vi "Test SFOAE Concurrent Stimuli.vi"() -> ()   [LabVIEW 2015]
uses:
  Typedefs/SFOAE-Stimulus Parameters.ctl
  Typedefs/SFOAE-Sweep Params.ctl
  <vilib>/Analysis/4window.llb/windowTd.ctl
  Utility VIs/Math VIs/FFT x(t) to dB,Degrees (1D).vi
  <vilib>/Analysis/NI_AALPro.lvlib
panel:
  out "Phase":cluster{"Array":dbl[], "Array":dbl[]}[](graph)
  out "Magnitude spectrum":cluster{"Array":dbl[], "Array":dbl[]}[](graph)
  in  "Cal File":path=path "C:/Experiment VIs/Cochlear Function Test Suite/LV Source/SFOAE VIs/Test VIs/dummy.calib"
  out "Waveform Graph":dbl[][](graph)
  in  "Fs (Hz)":dbl=100000.0
  in  "SFOAE Stim":T1={"Ear"=enum."Right", "Sweep"={"Type"=enum."Linear", "Fmin (kHz)"=4.0, "Fmax (kHz)"=14.25, "Rate"=5.0, "Ramp (ms)"=5.0, "Drain (ms)"=20.0}, "Suppressor"={"Delta"=50.0, "Ratio"=0.0, "Use ratio"=FALSE}, "Concurrent"={"Nsweeps"=1, "Overlap"=0.0}, "Ls (dB SPL)"=-23.0, "Lp (dB SPL)"={"Min"=-20.0, "Max"=-20.0, "Step"=5.0}}
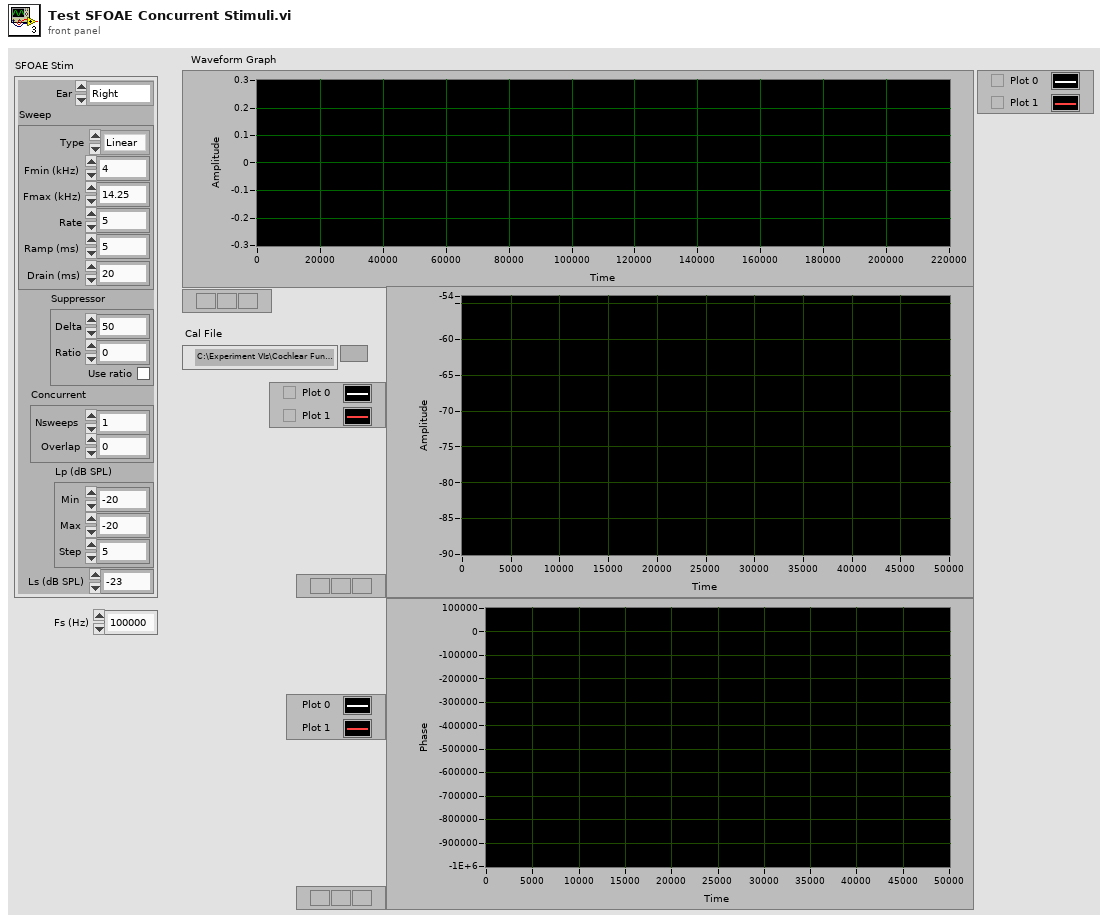
[diagram p1: front panel]
types:
  T1 = typedef "SFOAE-Stimulus Parameters.ctl" = cluster{"Ear":enum16{"Right", "Left"}, "Sweep":T2, "Suppressor":cluster{"Delta":dbl, "Ratio":dbl, "Use ratio":bool}, "Concurrent":cluster{"Nsweeps":i32, "Overlap":dbl}, "Ls (dB SPL)":dbl, "Lp (dB SPL)":cluster{"Min":dbl, "Max":dbl, "Step":dbl}}
  T2 = typedef "SFOAE-Sweep Params.ctl" = cluster{"Type":enum16{"Linear", "Log"}, "Fmin (kHz)":dbl, "Fmax (kHz)":dbl, "Rate":dbl, "Ramp (ms)":dbl, "Drain (ms)":dbl}
  T3 = typedef "NI_AALPro.lvlib/windowTd.ctl" = u32
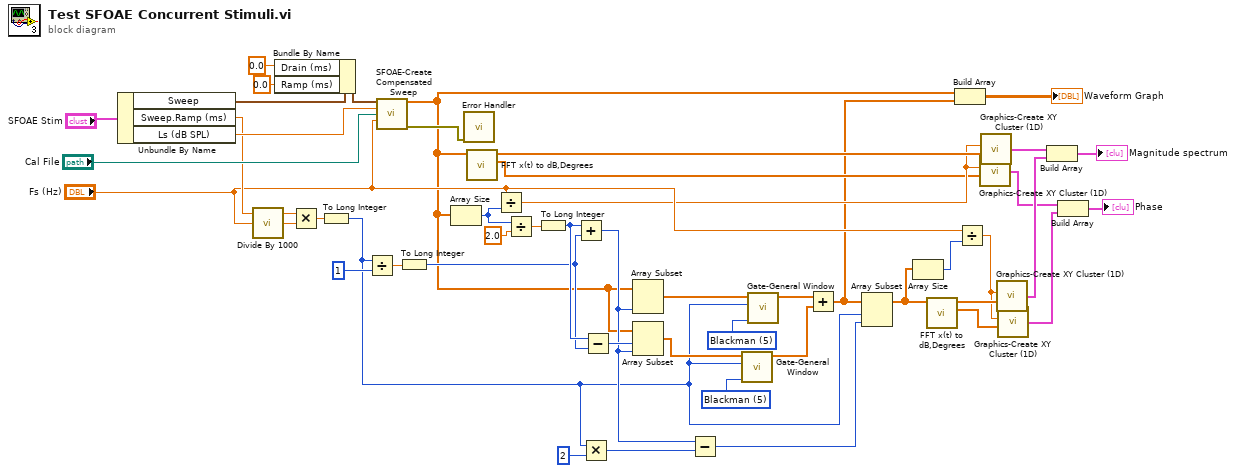
[diagram p0: block diagram]
diagram:
  w27 = T3 5 items=["Rectangle"=0, "Hanning"=1, "Hamming"=2, "Blackman-Harris"=3, "Exact Blackman"=4, "Blackman"=5, "Flat Top"=6, "4 Term B-Harris "=7, "7 Term B-Harris"=8, "Low Sidelobe"=9, "Blackman Nuttall"=11, "Triangle"=30, "Bartlett-Hanning"=31, "Bohman"=32, "Parzen"=33, "Welch"=34, "Kaiser"=60, "Dolph-Chebyshev"=61, "Gaussian"=62] ("window")
  w38 = T3 5 items=["Rectangle"=0, "Hanning"=1, "Hamming"=2, "Blackman-Harris"=3, "Exact Blackman"=4, "Blackman"=5, "Flat Top"=6, "4 Term B-Harris "=7, "7 Term B-Harris"=8, "Low Sidelobe"=9, "Blackman Nuttall"=11, "Triangle"=30, "Bartlett-Hanning"=31, "Bohman"=32, "Parzen"=33, "Welch"=34, "Kaiser"=60, "Dolph-Chebyshev"=61, "Gaussian"=62] ("window")
  n1 = Unbundle By Name("SFOAE Stim") -> ("Sweep"=w44:T2, "Sweep.Ramp (ms)"=w37:dbl, "Ls (dB SPL)"=w43:dbl)
  n2 = call "Divide By 1000.vi"("X"="Fs (Hz)") -> ("X/1000"=w36:dbl)
  n3 = Bundle By Name(cluster=w44, "Drain (ms)"=0.0, "Ramp (ms)"=0.0) -> (w40:T2)
  n4 = Multiply(x=w37, y=w36) -> (x*y=w35:dbl)
  n5 = To Long Integer(number=w35) -> (32bit integer=w5:i32)
  n6 = Divide(x=w5, y=1) -> (x/y=w30:dbl)
  n7 = call "SFOAE-Create Compensated Sweep.vi"("Sweep"=w40, "Level (dB SPL)"=w43, "Cal File"="Cal File", "Fs (Hz)"="Fs (Hz)") -> ("sweep"=w1:dbl[], "error out"=w41:errorcluster)  [unwired: 8 in, 2 out]
  n8 = To Long Integer(number=w30) -> (32bit integer=w28:i32)
  n9 = Array Size(array=w1) -> (size(s)=w34:i32)
  n10 = call "Error Handler.vi"("error in (no error)"=w41) -> ()  [unwired: 13 in, 2 out]
  n11 = call-poly "FFT x(t) to dB,Degrees.vi"("X"=w1) -> ("+Freq Phase of FFT (degrees)"=w19:dbl[], "+Freq. Mag of FFT (dB rms)"=w45:dbl[])  [unwired: 8 in, 1 out]
  n12 = Divide(x="Fs (Hz)", y=w34) -> (x/y=w20:dbl)
  n13 = Divide(x=w34, y=2.0) -> (x/y=w32:dbl)
  n14 = To Long Integer(number=w32) -> (32bit integer=w29:i32)
  n15 = Add(x=w29, y=w28) -> (x+y=w7:i32)
  n16 = Multiply(x=w5, y=2) -> (x*y=w6:i32)
  n17 = Subtract(x=w29, y=w28) -> (x-y=w22:i32)
  n18 = Array Subset(array=w1, length=w7) -> (w12:dbl[])  [unwired: 1 in]
  n19 = Array Subset(array=w1, index=w22, length=w7) -> (w11:dbl[])
  n20 = Subtract(x=w7, y=w6) -> (x-y=w3:i32)
  n21 = call "Gate-General Window.vi"("window"=w27, "Nramp"=w5, "X"=w11) -> ("X windowed"=w9:dbl[])  [unwired: 8 in]
  n22 = call "Gate-General Window.vi"("window"=w38, "Nramp"=w5, "X"=w12) -> ("X windowed"=w8:dbl[])  [unwired: 8 in]
  n23 = Add(x=w8, y=w9) -> (x+y=w10:dbl[])
  n24 = Array Subset(array=w10, index=w5, length=w3) -> (w2:dbl[])
  n25 = Array Size(array=w2) -> (size(s)=w24:i32)
  n26 = call-poly "FFT x(t) to dB,Degrees.vi"("X"=w2) -> ("+Freq Phase of FFT (degrees)"=w15:dbl[], "+Freq. Mag of FFT (dB rms)"=w26:dbl[])  [unwired: 8 in, 1 out]
  n27 = Build Array(w1, w10) -> (→"Waveform Graph":dbl[][])
  n28 = Divide(x="Fs (Hz)", y=w24) -> (x/y=w16:dbl)
  n29 = call "Graphics-Create XY Cluster (1D).vi"("Array"=w19, "dx"=w20) -> ("XY cluster"=w18:cluster{"Array":dbl[], "Array":dbl[]})  [unwired: 2 in]
  n30 = call "Graphics-Create XY Cluster (1D).vi"("Array"=w45, "dx"=w20) -> ("XY cluster"=w47:cluster{"Array":dbl[], "Array":dbl[]})  [unwired: 2 in]
  n31 = call "Graphics-Create XY Cluster (1D).vi"("Array"=w26, "dx"=w16) -> ("XY cluster"=w25:cluster{"Array":dbl[], "Array":dbl[]})  [unwired: 2 in]
  n32 = call "Graphics-Create XY Cluster (1D).vi"("Array"=w15, "dx"=w16) -> ("XY cluster"=w14:cluster{"Array":dbl[], "Array":dbl[]})  [unwired: 2 in]
  n33 = Build Array(w47, w25) -> (→"Magnitude spectrum":cluster{"Array":dbl[], "Array":dbl[]}[])
  n34 = Build Array(w18, w14) -> (→"Phase":cluster{"Array":dbl[], "Array":dbl[]}[])
